vi "readCommandTestHardpoint.vi"(8 "error in (no error)":errorcluster, 10 "Parser":refnum<class "U8ArrayParserAutoIndexing.lvclass">, 11 "M1M3SAL in":refnum<class "M1M3SAL.lvclass">) -> (0 "error out":errorcluster, 2 "CommandTestHardpoint":variant, 3 "M1M3SAL out":refnum<class "M1M3SAL.lvclass">)   [LabVIEW 2016, in "M1M3SupportCommunicator.lvlib" / "M1M3SAL.lvclass"]
uses:
  M1M3SAL.lvclass
  Common_RT_Utilities/U8ArrayParserAutoIndexing/U8ArrayParserAutoIndexing.lvclass
  DataTypes/Topics/CommandTestHardpoint.ctl
  DataTypes/Topics/Parts/CommandId.ctl
  DataTypes/Topics/M1M3SupportTopics.lvlib
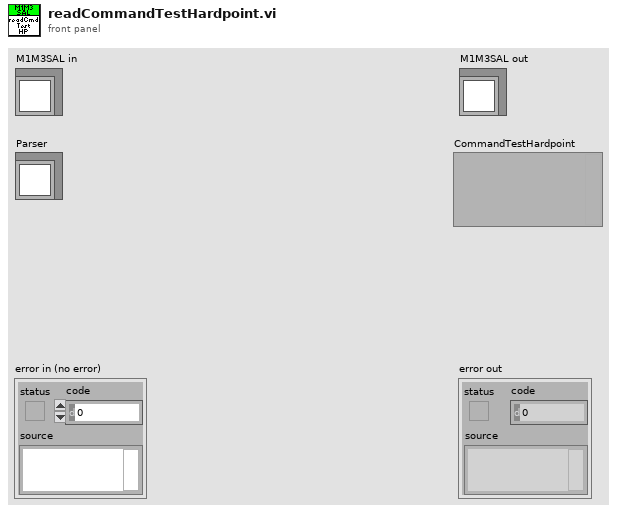
[diagram p1: front panel]
types:
  T1 = typedef "M1M3SupportTopics.lvlib/CommandTestHardpoint.ctl" = cluster{"CommandId":T2, "ActuatorId":i32}
  T2 = typedef "M1M3SupportTopics.lvlib/CommandId.ctl" = i32
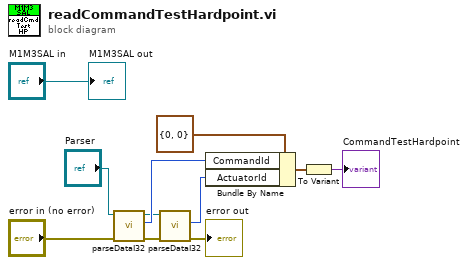
[diagram p0: block diagram]
diagram:
  n1 = call "parseDataI32.vi"("error in (no error)"="error in (no error)", "U8ArrayParserAutoIndexing in"="Parser") -> ("error out"=w4:errorcluster, "Data"=w6:i32, "U8ArrayParserAutoIndexing out"=w2:refnum<class "U8ArrayParserAutoIndexing.lvclass">)  [unwired: 7 in]
  n2 = call "parseDataI32.vi"("error in (no error)"=w4, "U8ArrayParserAutoIndexing in"=w2) -> ("error out"=→"error out":errorcluster, "Data"=w1:i32)  [unwired: 7 in, 1 out]
  n3 = Bundle By Name(cluster=T1 {"CommandId"=0, "ActuatorId"=0} ("CommandTestHardpoint"), "CommandId"=w6, "ActuatorId"=w1) -> (w10:T1)
  n4 = To Variant(anything=w10) -> (Variant=→"CommandTestHardpoint":variant)
  "M1M3SAL out" <- "M1M3SAL in"
